vi "Write Input Values.vi"(8 "error in (no error)":errorcluster, 10 "Cluster":T1, 11 "Mode in":refnum<class "Mode.lvclass">) -> (0 "error out":errorcluster, 3 "Mode out":refnum<class "Mode.lvclass">)   [LabVIEW 2023, in "Mode.lvclass"]
uses:
  Mode.lvclass
  Typedef/Input Values.ctl
  Mode.lvclass/Mode.ctl
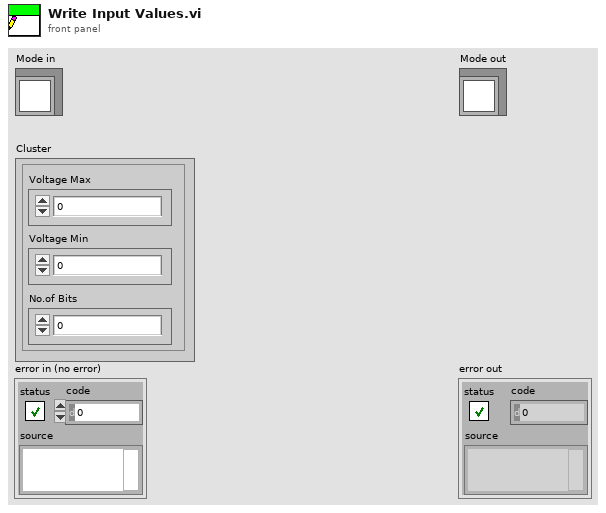
[diagram p1: front panel]
types:
  T1 = typedef "Input Values.ctl" = cluster{"Voltage Max":dbl, "Voltage Min":dbl, "No.of Bits":i32}
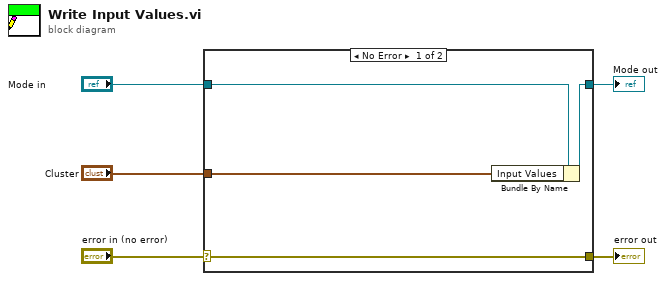
[diagram p0: block diagram]
diagram:
  n1 = case shown="No Error" "error in (no error)" {
    selector: "error in (no error)" -> [w9 w10]
    tunnel: [w9 w10] -> w4
    tunnel: [w7 w11] -> w2
    tunnel: "Mode in" -> [w8 w11]
    tunnel: "Cluster" -> [w6 _]
    frame No Error {
      n2 = Bundle By Name(cluster=w8, "Input Values"=w6) -> (w7:refnum<class "Mode.lvclass">)
    }
    frame Error {
    }
  }
  "error out" <- w4
  "Mode out" <- w2
